vi "Supply_SetVolts.vi"(8 "error in (no error)":errorcluster, 9 "Command string":string, 10 "Volts IN [V]":dbl, 11 "SupplyControl in":refnum<class "SupplyControl.lvclass">) -> (0 "error out":errorcluster, 2 "Compliance exceeded?":bool, 3 "SupplyControl out":refnum<class "SupplyControl.lvclass">)   [LabVIEW 2018, in "SupplyControl.lvclass"]
uses:
  SupplyControl.lvclass
  C:/Users/Graham Greig/Desktop/itk-strip-sensor-qc-master/itk-strip-sensor-qc-master/InstrControl/InstrControl.lvclass
  InstrControl.lvclass
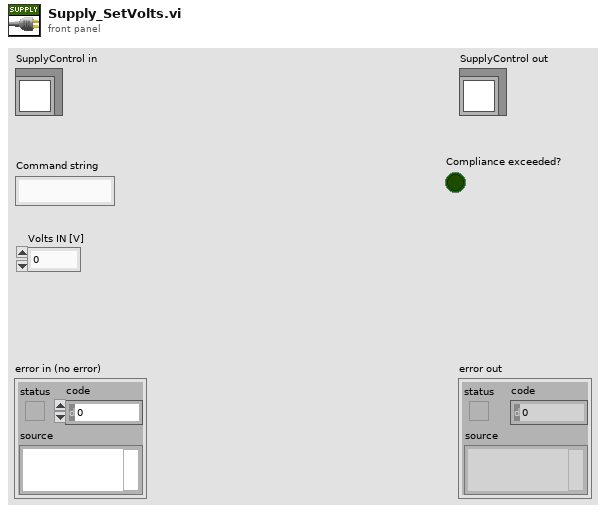
[diagram p1: front panel]
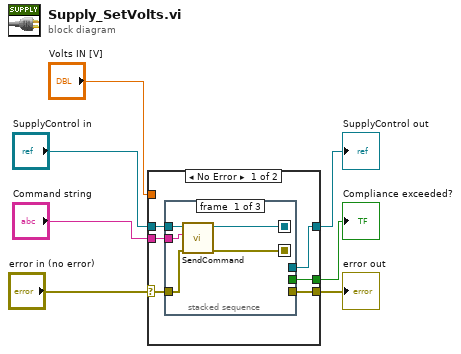
[diagram p0: block diagram]
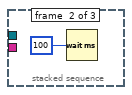
[diagram p2: hidden frame]
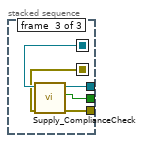
[diagram p3: hidden frame]
diagram:
  n1 = case shown="No Error" "error in (no error)" {
    selector: "error in (no error)" -> [w10 w26]
    tunnel: [w11 w26] -> w6
    tunnel: [w13 w25] -> w4
    tunnel: "SupplyControl in" -> [w9 w25]
    tunnel: [w12 _] -> w3
    tunnel: "Command string" -> [w8 _]
    tunnel: "Volts IN [V]" -> [_ _]
    frame No Error {
      n2 = stacked-sequence {
        seq-local: [w17 _ _] -> [_ _ w20]
        seq-local: [w16 _ _] -> [_ _ w21]
        tunnel: [_ _ w24] -> w13
        tunnel: [_ _ w23] -> w12
        tunnel: [_ _ w22] -> w11
        tunnel: w10 -> [w18 _ _]
        tunnel: w9 -> [w15 _ _]
        tunnel: w8 -> [w14 _ _]
        frame #0 {
          n3 = call "SendCommand.vi"("error in (no error)"=w18, "Command string"=w14, "InstControl in"=w15) -> ("error out"=w17:errorcluster, "InstControl out"=w16:refnum<class "SupplyControl.lvclass">)  [unwired: 7 in]
        }
        frame #1 {
          n4 = Wait (ms)(milliseconds to wait=u32 100) -> ()  [unwired: 1 out]
        }
        frame #2 {
          n5 = call-dynamic "Supply_ComplianceCheck.vi"("error in (no error)"=w20, "SupplyControl in"=w21) -> ("error out"=w22:errorcluster, "Compliance exceeded?"=w23:bool, "SupplyControl out"=w24:refnum<class "SupplyControl.lvclass">)  [unwired: 6 in, 1 out]
        }
      }
    }
    frame Error {
    }
  }
  "error out" <- w6
  "SupplyControl out" <- w4
  "Compliance exceeded?" <- w3
